vi "Query Pulse Waveform.vi"(8 "error in (no error)":errorcluster, 10 "Channel (0: Channel 1)":T1 items=["Channel 1", "Channel 2"], 11 "VISA resource name":refnum<visa-resource-name>) -> (0 "Delay":dbl[unit], 1 "Trailing":dbl[unit], 2 "Leading":dbl[unit], 3 "Duty Cycle":dbl, 4 "error out":errorcluster, 5 "VISA resource name out":refnum<visa-resource-name>)   [LabVIEW 2009, in "Tektronix AFG 3000 Series.lvlib"]
uses:
  Tektronix AFG 3000 Series.lvlib
  controls.llb/Channel.ctl
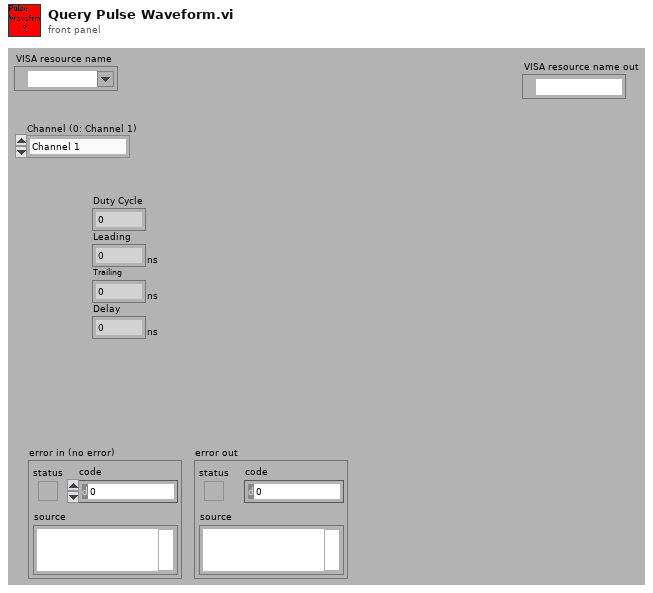
[diagram p1: front panel]
types:
  T1 = typedef "Channel.ctl" = u16
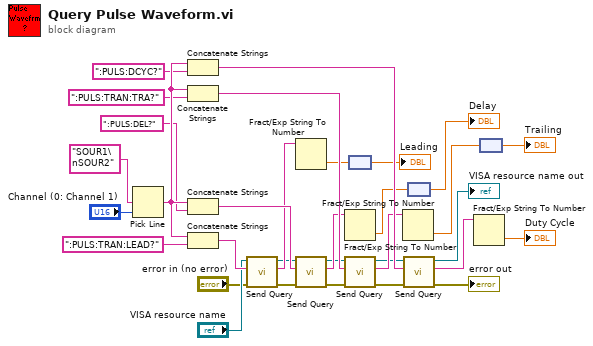
[diagram p0: block diagram]
diagram:
  n1 = Pick Line(multi-line string="SOUR1\nSOUR2" ("string (\"\")"), line index="Channel (0: Channel 1)") -> (output string=w30:string)  [unwired: 1 out]
  n2 = Concatenate Strings(w30, ":PULS:DCYC?") -> (w22:string)
  n3 = Concatenate Strings(w30, ":PULS:TRAN:TRA?") -> (w23:string)
  n4 = Concatenate Strings(w30, ":PULS:DEL?") -> (w24:string)
  n5 = Concatenate Strings(w30, ":PULS:TRAN:LEAD?") -> (w25:string)
  n6 = call "Send Query.vi"("error in (no error)"="error in (no error)", "write buffer"=w25, "VISA resource name"="VISA resource name") -> ("error out"=w4:errorcluster, "read buffer"=w18:string, "VISA resource name out"=w9:refnum<visa-resource-name>)  [unwired: 1 in, 5 out]
  n7 = Fract/Exp String To Number(string=w18) -> (number=w16:dbl)  [unwired: 4 out]
  n8 = call "Send Query.vi"("error in (no error)"=w4, "write buffer"=w24, "VISA resource name"=w9) -> ("error out"=w3:errorcluster, "read buffer"=w19:string, "VISA resource name out"=w8:refnum<visa-resource-name>)  [unwired: 1 in, 5 out]
  n9 = Fract/Exp String To Number(string=w19) -> (number=w14:dbl)  [unwired: 4 out]
  n10 = call "Send Query.vi"("error in (no error)"=w3, "write buffer"=w23, "VISA resource name"=w8) -> ("error out"=w2:errorcluster, "read buffer"=w20:string, "VISA resource name out"=w7:refnum<visa-resource-name>)  [unwired: 1 in, 5 out]
  n11 = node(w16) -> (→"Leading":dbl[unit])
  n12 = Fract/Exp String To Number(string=w20) -> (number=w13:dbl)  [unwired: 4 out]
  n13 = call "Send Query.vi"("error in (no error)"=w2, "write buffer"=w22, "VISA resource name"=w7) -> ("error out"=→"error out":errorcluster, "read buffer"=w21:string, "VISA resource name out"=→"VISA resource name out":refnum<visa-resource-name>)  [unwired: 1 in, 5 out]
  n14 = node(w14) -> (→"Delay":dbl[unit])
  n15 = Fract/Exp String To Number(string=w21) -> (number=→"Duty Cycle":dbl)  [unwired: 4 out]
  n16 = node(w13) -> (→"Trailing":dbl[unit])
